vi "AMI_SetCampo Y axis.vi"(6 "error in (no error)":errorcluster, 7 "Index":i8) -> (0 "error out":errorcluster, 3 "resulting string Y":string="Set Magnetic Field 1000.000Tesla at 100.000Tesla/min, Linear, Persistent, Sweep&meas")   [LabVIEW 2017]
doc: "Use this template to create a dialog box. This template polls the state of the buttons on the front panel and does not use events. Use the Dialog Using Events template (not available in Base package) to create a dialog box with event handling."
panel:
  in  "Modo Rampa":u16(ring) items=["RAMP", "PAUSE", "MANUAL UP", "MANUAL DOWN", "ZERO"]
  out "Y Ramp Units":u16(ring)=1 items=["Per SECOND", "Per MINUTE"]
  out "Y Field Units":u16(ring)=1 items=["KGauss", "Tesla"]
  out "Wait stability":bool=TRUE
  in  "Field Mode":i32(ring) items=["Persistent", "Driven"]
  in  "Approach":i32(ring) items=["Linear", "NoOvershoot", "Oscillate"]
  in  "Y rate":dbl=0.03 min=0.0 max=0.1 format="%.3f"
  in  "Y target":dbl=0.1 min=-0.5 max=0.5 format="%.3f"
  out "Cancelled?":bool
  in  "Cancel":bool
  in  "OK":bool
  # "Y AXIS MAGNETIC FIELD"
  # "Junio 2022 V2.0  a-sslcdms"
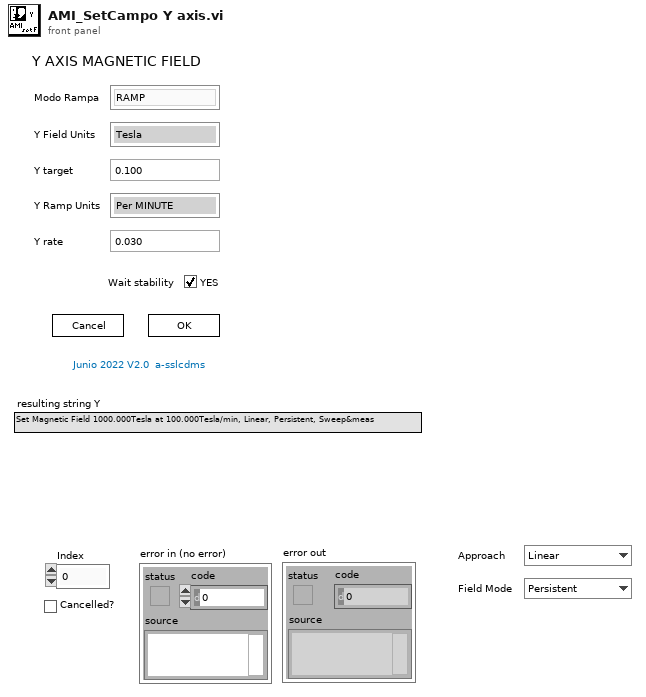
[diagram p1: front panel]
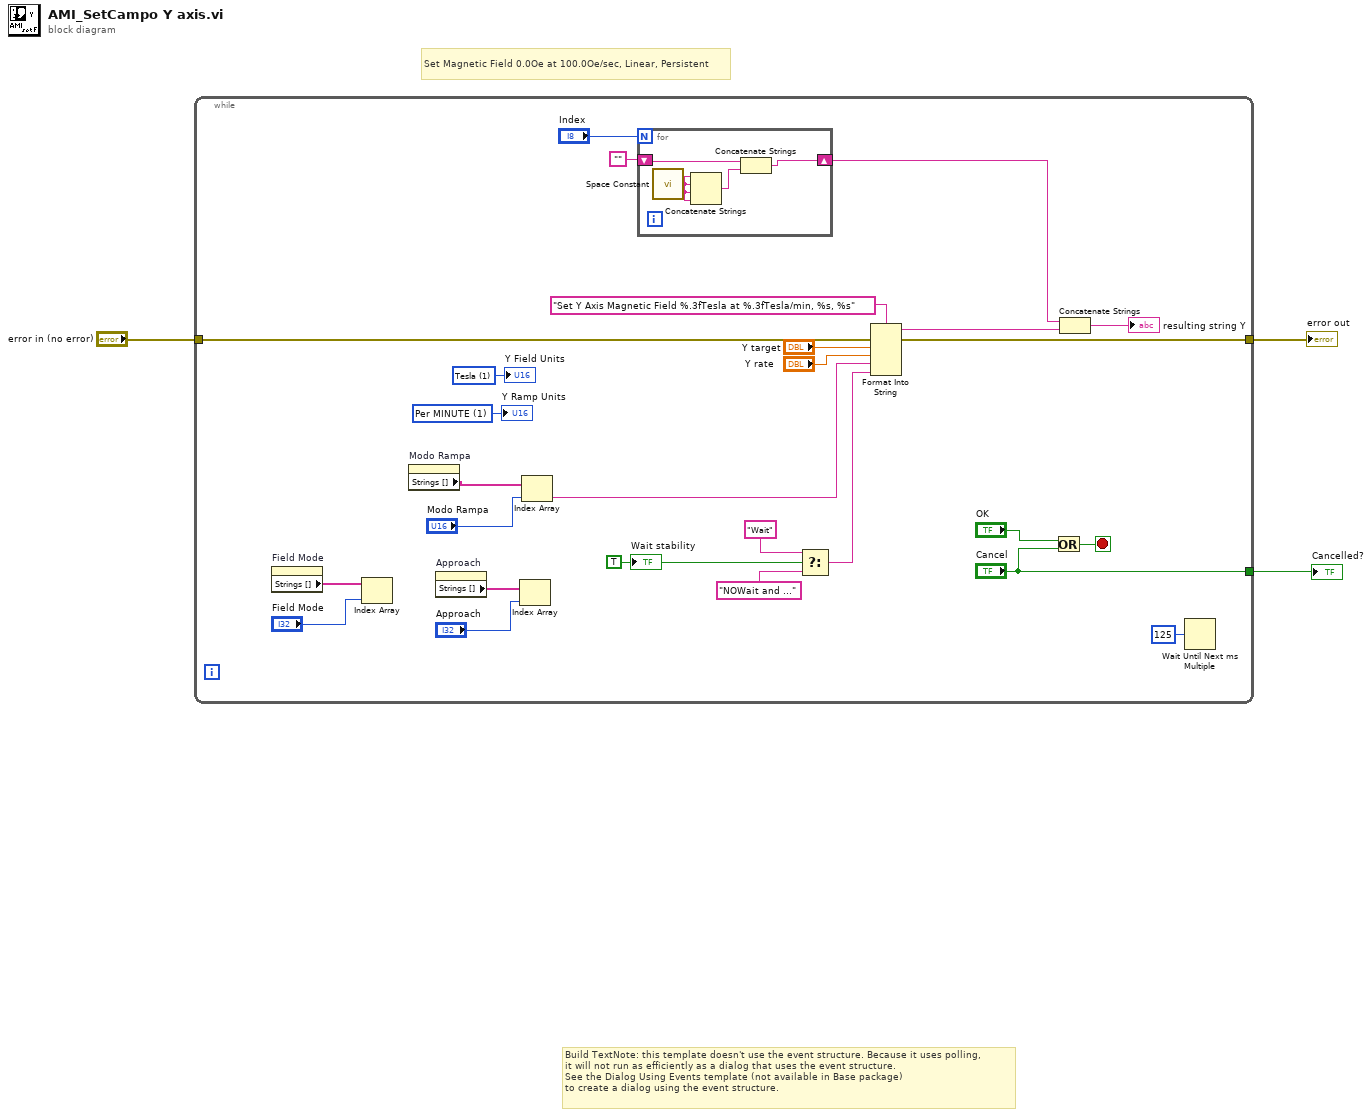
[diagram p0: block diagram]
diagram:
  # "Set Magnetic Field 0.0Oe at 100.0Oe/sec, Linear, Persistent"
  # "Build TextNote: this template doesn't use the event structure. Because it uses polling, \nit will not run as efficiently as a dialog that uses the event structure.\nSee the Dialog Using Events template (not available in Base package) \nto create a dialog using the event structure."
  n1 = while {
    tunnel: ["Cancel"] -> w3
    tunnel: [w8] -> w2
    tunnel: "error in (no error)" -> [w10]
    stop <- w29 stop-if-true
    w11 = u16 1 items=["Per SECOND", "Per MINUTE"] ("Ramp Units")
    w12 = u16 1 items=["KGauss", "Tesla"] ("Field Units")
    w15 = TRUE ("Wait stability")
    n2 = property on="Field Mode" class="Ring (strict)"() -> ("Strings []"=w18:string[])  [unwired: 2 in, 2 out]
    n3 = Index Array(array=w18, index="Field Mode") -> ()  [unwired: 1 out]
    n4 = property on="Modo Rampa" class="Ring (strict)"() -> ("Strings []"=w5:string[])  [unwired: 2 in, 2 out]
    n5 = property on="Approach" class="Ring (strict)"() -> ("Strings []"=w21:string[])  [unwired: 2 in, 2 out]
    n6 = Index Array(array=w21, index="Approach") -> ()  [unwired: 1 out]
    n7 = Index Array(array=w5, index="Modo Rampa") -> (element=w4:string)
    n8 = for {
      N: "Index" -> [_]
      shift-right: [w33] -> w9
      shift-left: "" -> [w32]
      n9 = call <vilib>:"Space Constant.vi"() -> ("String"=w31:string)
      n10 = Concatenate Strings(w31, w31, w31, w31) -> (w34:string)
      n11 = Concatenate Strings(w32, w34) -> (w33:string)
    }
    n12 = Select(t="Wait", s=w15, f="NOWait and ...") -> (s? t:f=w7:string)
    n13 = Format Into String(format string="Set Y Axis Magnetic Field %.3fTesla at %.3fTesla/min, %s, %s", error in=w10, "Y target", "Y rate", w4, w7) -> (resulting string=w23:string, error out=w8:errorcluster)  [unwired: 1 in]
    n14 = Or(x="OK", y="Cancel") -> (x .or. y?=w29:bool)
    n15 = Concatenate Strings(w9, w23) -> (→"resulting string Y":string)
    n16 = Wait Until Next ms Multiple(millisecond multiple=u32 125) -> ()  [unwired: 1 out]
    "Wait stability" <- w15
    "Y Field Units" <- w12
    "Y Ramp Units" <- w11
  }
  "Cancelled?" <- w3
  "error out" <- w2
